vi "Disconnect.vi"(8 "error in (no error)":errorcluster, 11 "TCP Stream in":refnum<class "TCP Stream.lvclass">) -> (0 "error out":errorcluster, 3 "TCP Stream out":refnum<class "TCP Stream.lvclass">)   [LabVIEW 2020, in "TCP Stream.lvclass"]
uses:
  TCP Stream.lvclass
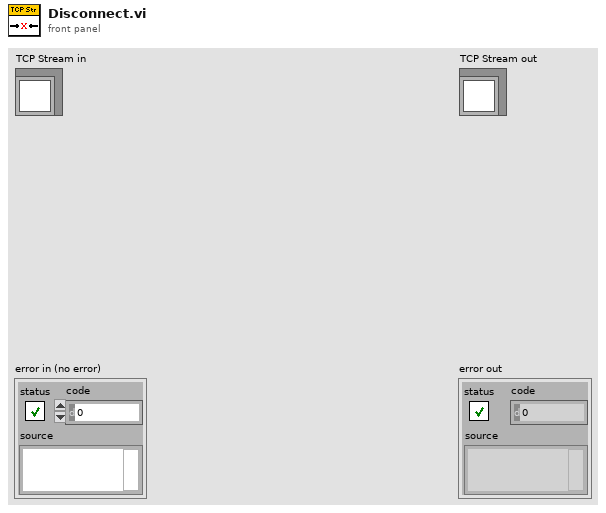
[diagram p1: front panel]
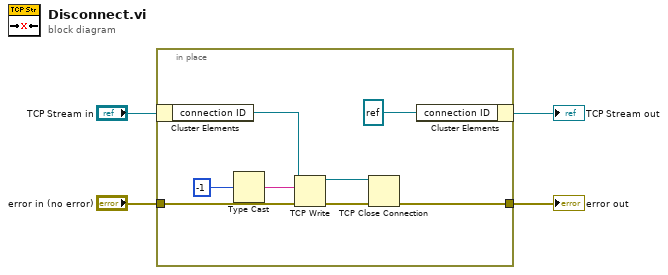
[diagram p0: block diagram]
diagram:
  n1 = in-place {
    in-place-border: "error in (no error)" -> [w9]
    in-place-border: [w5] -> w2
    n2 = in-place-cluster #1("TCP Stream in") -> ("connection ID"=w10:refnum<k5>)
    n3 = Type Cast(x=-1 ("bytes to read")) -> (*(type *) &x=w12:string)  [unwired: 1 in]
    n4 = TCP Write(connection ID=w10, data in=w12, error in (no error)=w9) -> (connection ID out=w7:refnum<k5>, error out=w8:errorcluster)  [unwired: 1 in, 1 out]
    n5 = TCP Close Connection(connection ID=w7, error in (no error)=w8) -> (error out=w5:errorcluster)  [unwired: 1 in, 1 out]
    n6 = in-place-cluster #1("connection ID"=refnum<k5> refnum) -> (→"TCP Stream out":refnum<class "TCP Stream.lvclass">)
  }
  "error out" <- w2
